vi "ConfigInstr.vi"(6 "InstrumentName":string, 7 "VisaRessIn":refnum<visa-resource-name>, 8 "error in (no error)":errorcluster caption="entrée d'erreur (pas d'erreur)", 9 "FirstClassInst":bool, 10 "Function":string, 11 "GenData In":refnum<class "LeafMagnetometer.lvclass"> caption="DNL_LabVIEW Object in") -> (0 "error out":errorcluster caption="sortie d'erreur", 3 "GenData Out":refnum<class "LeafMagnetometer.lvclass"> caption="DNL_LabVIEW Object out")   [LabVIEW 2010, in "LeafMagnetometer.lvclass"]
uses:
  LeafMagnetometer.lvclass
  LeafMagnetometer_Func.ctl
  LeafMagnetometer.lvclass/LeafMagnetometer.ctl
  BaseDevice/BaseDevice.lvclass
panel:
  in  "DefaultDev_Func":T1
  out "VisaRessOut":refnum<visa-resource-name>
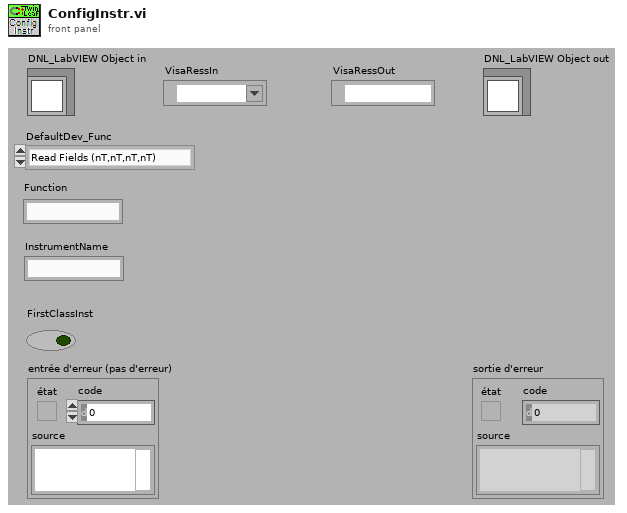
[diagram p1: front panel]
types:
  T1 = typedef "LeafMagnetometer.lvclass/LeafMagnetometer_Func.ctl" = enum16{"Read Fields (nT,nT,nT,nT)"}
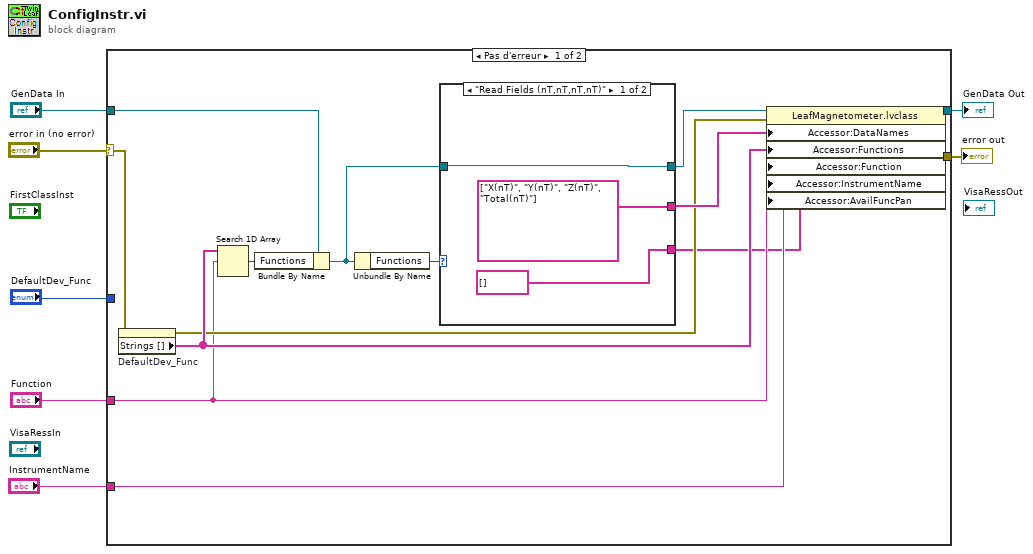
[diagram p0: block diagram]
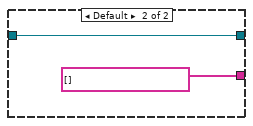
[diagram p2: hidden frame]
diagram:
  n1 = case shown="Pas d'erreur" "error in (no error)" {
    selector: "error in (no error)" -> [w14 w28]
    tunnel: [w21 w28] -> w6
    tunnel: "GenData In" -> [w15 w27]
    tunnel: [w20 w27] -> w4
    tunnel: "DefaultDev_Func" -> [_ _]
    tunnel: "Function" -> [w10 _]
    tunnel: "InstrumentName" -> [w9 _]
    frame No Error {
      n2 = property on="DefaultDev_Func" class="Énum (strict)"(error in=w14) -> (error out=w13:errorcluster, "Strings []"=w17:string[])  [unwired: 1 in, 1 out]
      n3 = Search 1D Array(1D array=w17, element=w10) -> (index of element=w16:i32)  [unwired: 1 in]
      n4 = Bundle By Name(cluster=w15, "Functions"=w16) -> (w12:refnum<class "LeafMagnetometer.lvclass">)
      n5 = Unbundle By Name(w12) -> ("Functions"=w18:T1)
      n6 = case shown="\"Read Fields (nT,nT,nT,nT)\"" w18 {
        tunnel: [string[] ["X(nT)", "Y(nT)", "Z(nT)", "Total(nT)"] string[] []] -> w19
        tunnel: w12 -> [w24 w25]
        tunnel: [w24 w25] -> w11
        tunnel: [string[] [] _] -> w8
        frame "Read Fields (nT,nT,nT,nT)" {
        }
        frame Default {
        }
      }
      n7 = property class="LeafMagnetometer.lvclass"(reference=w11, error in=w13, "Accessor:DataNames"=w19, "Accessor:Functions"=w17, "Accessor:Function"=w10, "Accessor:InstrumentName"=w9, "Accessor:AvailFuncPan"=w8) -> (reference out=w20:refnum<class "LeafMagnetometer.lvclass">, error out=w21:errorcluster)
    }
    frame Error {
    }
  }
  "error out" <- w6
  "GenData Out" <- w4
